vi "convert V to d.vi"(8 "error in (no error)":errorcluster, 10 "V_strain (V)":dbl) -> (0 "error out":errorcluster, 1 "C (pF)":dbl, 2 "d (um)":dbl)   [LabVIEW 2019, in "Inst.RP100.lvlib" / "Inst.RP100.lvclass"]
doc: "This VI will convert a voltage applied to the strain cell to expected capacitance and to an expected displacment. Conversion is based on calibration by Razorbill of capacitance vs displacement at 300K, converting the calibration to values at 4K, and by measurements by us of capacitance vs voltage us at 50 mK.\n\nShould be reliable in the range -140 V ... +130 V."
uses:
  Inst.RP100.lvclass
panel:
  out "our measurements <50 mK":cluster{dbl[], dbl[]}[](graph)
  out "convert measured C to expected d":cluster{dbl[], dbl[]}(graph)
  out "calibration from Razorbill":cluster{"all rows":dbl[], "all rows":dbl[]}[](graph)
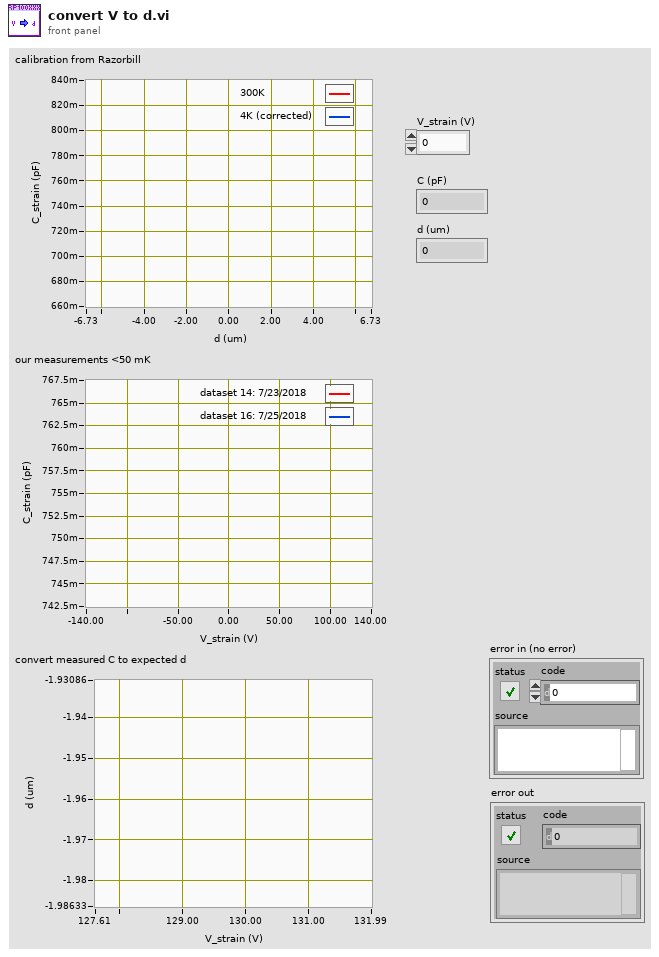
[diagram p1: front panel]
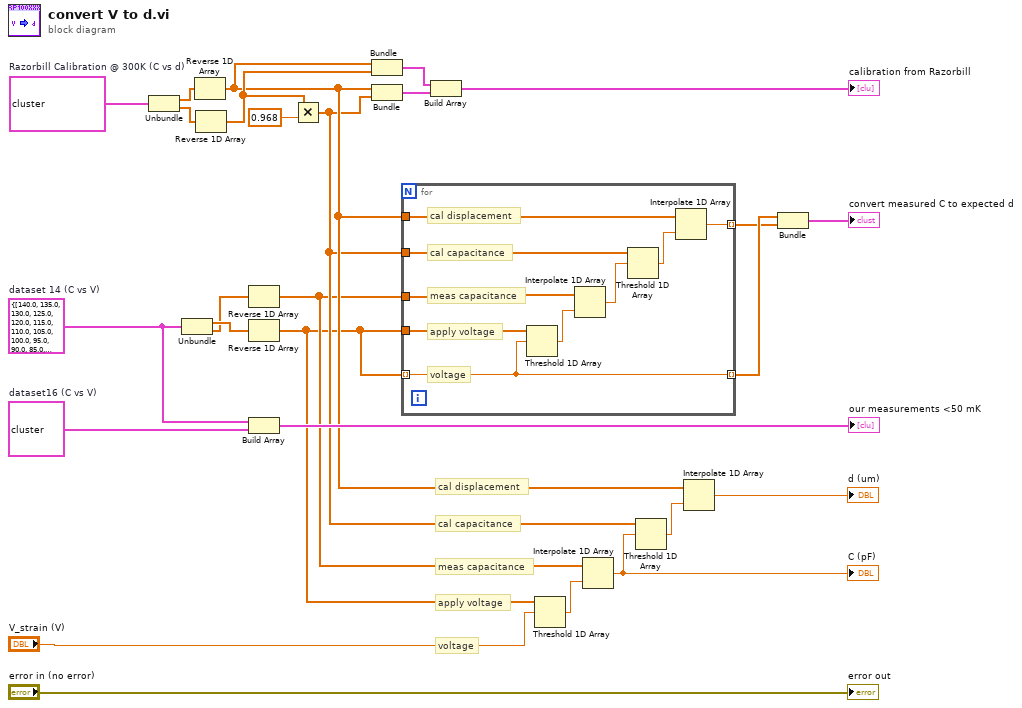
[diagram p0: block diagram]
diagram:
  w18 = cluster{dbl[], dbl[]} {array[987 elements], array[987 elements]}  # dataset16 (C vs V)
  w12 = cluster{dbl[], dbl[]} {[140.0, 135.0, 130.0, 125.0, 120.0, 115.0, 110.0, 105.0, 100.0, 95.0, 90.0, 85.0, 80.0, 75.0, 70.0, 65.0, 60.0, 55.0, 50.0, 45.0, 40.0, 35.0, 30.0, 25.0, 20.0, 15.0, 10.0, 5.0, 0.0, -5.0, -10.0, -15.0, -20.0, -25.0, -30.0, -35.0, -40.0, -45.0, -50.0, -55.0, -60.0, -65.0, -70.0, -75.0, -80.0, -85.0, -90.0, -95.0, -100.0, -105.0, -110.0, -115.0, -120.0, -125.0, -130.0, -135.0, -140.0], [0.75086, 0.74594, 0.74364, 0.74399, 0.74427, 0.74472, 0.74509, 0.74541, 0.74575, 0.746, 0.74625, 0.74658, 0.74691, 0.7473, 0.74773, 0.74809, 0.74842, 0.74876, 0.74909, 0.74944, 0.74978, 0.75017, 0.7506, 0.75099, 0.75141, 0.75177, 0.75204, 0.75244, 0.75278, 0.75325, 0.75365, 0.75411, 0.75455, 0.75494, 0.7553, 0.75566, 0.75599, 0.75638, 0.75685, 0.75732, 0.75778, 0.75825, 0.75871, 0.75909, 0.75947, 0.75987, 0.76027, 0.76073, 0.76126, 0.7618, 0.76235, 0.76284, 0.76328, 0.76376, 0.7642, 0.76462, 0.76508]}  # dataset 14 (C vs V)
  w24 = cluster{"all rows":dbl[], "all rows":dbl[]} {"all rows"=[-6.729466796998171, -6.6508615753295075, -6.562134809022304, -6.484100964873558, -6.406230371444788, -6.327053772256207, -6.245428412267978, -6.164619305879633, -6.075647663492464, -5.989328845304913, -5.9083156755165955, -5.831383773727691, -5.741916548797737, -5.656093313152971, -5.573161947404931, -5.487210443337327, -5.407135965188876, -5.323572002900927, -5.260210317210065, -5.171136643122911, -5.101740511175776, -5.011486184560221, -4.930851989657564, -4.843104727670219, -4.763928128481638, -4.679854007693763, -4.589599681078207, -4.489585293561203, -4.405103045973387, -4.322334930945324, -4.245373877242137, -4.141126631771457, -4.0492981017847, -3.9599183325975904, -3.8688244308507285, -3.7909538374219585, -3.697084673435496, -3.6146430598473858, -3.5308954404994637, -3.4603711294696344, -3.379562023081289, -3.2816115910954142, -3.1942724559080116, -3.111947449977026, -3.0195941855332027, -2.9417235921044327, -2.849813436757688, -2.7673718231695776, -2.691949990540455, -2.604004495535995, -2.5200469824052467, -2.4404622564167235, -2.36393848142776, -2.2797186010684785, -2.205626095730592, -2.114532193983729, -2.0517214794727874, -1.9682595488848245, -1.8890829496962427, -1.7870512497109576, -1.7036913508229805, -1.6311468121334425, -1.5503377057450969, -1.4621823169578096, -1.3532124613735252, -1.2834227785835903, -1.2004710064955528, -1.1193558050072507, -1.0401792058186707, -0.9678824584005259, -0.8818260074415072, -0.8010169010531616, -0.7172692817052386, -0.6449084000756766, -0.555441175145722, -0.44545683294443883, -0.3574851012171276, -0.28126742132811877, -0.16831832944440883, -0.07832637005738796, 0.0019317651510384337, 0.08347549977927926, 0.1613460932080475, 0.2550111937945392, 0.33602436358285637, 0.41038506653213247, 0.4835330498472974, 0.5771456769880814, 0.6785243740934614, 0.759333480481807, 0.8489581257488812, 0.9337552140109366, 1.0208611338840896, 1.1071799520716414, 1.1873768682600758, 1.268430850728386, 1.3416487986378272, 1.4322529482247592, 1.5235567437544475, 1.6159100081982736, 1.695494734186795, 1.782775565545636, 1.8744991486409806, 1.9575121397490083, 2.041994387336823, 2.113008450526582, 2.1990211736141774, 2.306460553698683, 2.382372138487735, 2.460732484076434, 2.5424598757646475, 2.6208814403733367, 2.7094566167262784, 2.7871173163722194, 2.8826189875584465, 2.9602796872043893, 3.0282327993945906, 3.1316929431796687, 3.2115225452481564, 3.2884136343570685, 3.3746100145046363, 3.4556290146758073, 3.543390852620295, 3.623893863908684, 3.712539004855902, 3.7914590671988044, 3.90335869016838, 3.986004367156461, 4.064670807845117, 4.144867724033551, 4.226595115721764, 4.329836620149731, 4.4111704609951445, 4.494183452103172, 4.574992558491518, 4.679309768556475, 4.7582823043450855, 4.837989468373589, 4.9196381498932436, 4.991002036054379, 5.095293009396482, 5.174659096027893, 5.263863953729313, 5.335883757961785, 5.42618181244876, 5.509439679636754, 5.5902487860251, 5.670323264173552, 5.744520716402851, 5.835124865989785, 5.914301465178367, 5.993559689726936, 6.080000945954469, 6.158667386643124, 6.255821971369111, 6.3156941729204785, 6.413950700006309, 6.49567809169452, 6.576854512202816, 6.655459733871476, 6.732595699060353], "all rows"=[0.8239726046128422, 0.8233546085808581, 0.8220124405329421, 0.821121504950495, 0.8201087172717272, 0.8191494340545165, 0.8182629859430387, 0.8172025620339811, 0.816289534286762, 0.8151667172717272, 0.8141683412785723, 0.8133687084708471, 0.8122323180889517, 0.8110619757975797, 0.8099146675467546, 0.8088083678767877, 0.8081422891089108, 0.8074302310231023, 0.8064992533920058, 0.8054477612761276, 0.8044211598302687, 0.803141195033789, 0.8024719207920792, 0.8011270602615816, 0.8001826202175772, 0.7993811874901775, 0.7979858305830583, 0.7972837139713971, 0.7960217680968097, 0.7950810561056105, 0.7941823290900518, 0.7929995599559956, 0.791969167583425, 0.7909528589658965, 0.7895666446644665, 0.7888343485777148, 0.7875887055372204, 0.7869344134413441, 0.7860358679867987, 0.7850114301430142, 0.7841143674367437, 0.7831616428309497, 0.7820587605427209, 0.7809921232123211, 0.7801618547854785, 0.7793579933993399, 0.7781391272460579, 0.7772174697469747, 0.7763693377337733, 0.7753689768976897, 0.774542591859186, 0.7735318753208653, 0.7730381672167216, 0.7717030583058305, 0.7706902706270626, 0.769913592959296, 0.7691769141914191, 0.7683409069795868, 0.7675179738418286, 0.7665459185918592, 0.7656993399339933, 0.7649476571657166, 0.7637281320132012, 0.763066402640264, 0.7619324532453244, 0.76118166483315, 0.7602509460946094, 0.7592192592592593, 0.7584995379537953, 0.7577761181832469, 0.7566159836555084, 0.7559636853685369, 0.7553095674367436, 0.7545268316831683, 0.7536930127298443, 0.7524911595159516, 0.7516026402640263, 0.7507677117711771, 0.7494978437843784, 0.7486007810781078, 0.7475720160301744, 0.7463821680339462, 0.745556204620462, 0.7449387458745874, 0.7439622031536487, 0.7430681953795379, 0.7422603174603174, 0.7408099273927392, 0.7399338349834983, 0.7389769680968097, 0.7378461254125412, 0.7370898632720415, 0.7363176237623762, 0.7354648316831682, 0.7346054809925437, 0.7339969108910891, 0.7333662486248624, 0.7321080308030803, 0.7311915511551155, 0.7302928241395568, 0.7296226622662266, 0.7287305924878202, 0.7276871815181518, 0.7267644884488449, 0.7260787930221593, 0.725368539787312, 0.7245587238723872, 0.7236156152758133, 0.7229932868842439, 0.722025201320132, 0.7213471617161715, 0.7204361188118812, 0.7197943611504007, 0.7191552663837812, 0.717850447901933, 0.7170560176017602, 0.7166521452145214, 0.7153421488815548, 0.7147632651265126, 0.7141495171739396, 0.7132347634763476, 0.7124181423856671, 0.7118056765676567, 0.7111132252780833, 0.7099043696369637, 0.709133905390539, 0.7082290759075907, 0.7075300660066006, 0.7066174697469747, 0.7059883608360835, 0.7052077997799779, 0.7042430551626591, 0.7035231859185919, 0.7028412629262927, 0.7019822574257426, 0.7010927026035936, 0.7004312321232123, 0.6996149438943894, 0.6989039509665251, 0.6982604180418042, 0.6972157865786579, 0.6964940311173975, 0.6957484205563413, 0.6950954565456545, 0.6943097176384305, 0.6935175064173084, 0.692731602760276, 0.6922194191419142, 0.691411846962474, 0.6907249187140936, 0.6900152079207921, 0.689380196259626, 0.6885364136413641, 0.6878995379537953, 0.6871383938393839, 0.6867034543454344, 0.6857485291529153, 0.6849986468646864, 0.6842938895489549, 0.6839582518251826, 0.6833031595159516]}  # Razorbill Calibration @ 300K (C vs d)
  # "cal displacement"
  # "cal capacitance"
  # "meas capacitance"
  # "apply voltage"
  # "voltage"
  n1 = Unbundle(w24) -> ("all rows"=w21:dbl[], "all rows"=w22:dbl[])
  n2 = Unbundle(w12) -> (w14:dbl[], w13:dbl[])
  n3 = Reverse 1D Array(array=w21) -> (reversed array=w7:dbl[])
  n4 = Reverse 1D Array(array=w22) -> (reversed array=w20:dbl[])
  n5 = Reverse 1D Array(array=w13) -> (reversed array=w5:dbl[])
  n6 = Reverse 1D Array(array=w14) -> (reversed array=w4:dbl[])
  n7 = Build Array(w12, w18) -> (→"our measurements <50 mK":cluster{dbl[], dbl[]}[])
  n8 = Multiply(x=w20, y=0.968) -> (x*y=w6:dbl[])
  n9 = Bundle(w7, w20) -> (w19:cluster{dbl[], dbl[]})  [unwired: 1 in]
  n10 = Bundle(w7, w6) -> (w25:cluster{dbl[], dbl[]})  [unwired: 1 in]
  n11 = for {
    tunnel: w4 -> [w27] mode=indexing
    tunnel: w4 -> [w35]
    tunnel: w5 -> [w33]
    tunnel: w6 -> [w30]
    tunnel: w7 -> [w29]
    tunnel: [w28] -> w16 mode=indexing
    tunnel: [w27] -> w17 mode=indexing
    # "cal displacement"
    # "cal capacitance"
    # "meas capacitance"
    # "apply voltage"
    # "voltage"
    n12 = Threshold 1D Array(2:w27, 3:w35) -> (0:w34:dbl)  [unwired: 1 in]
    n13 = Interpolate 1D Array(1:w34, 2:w33) -> (0:w31:dbl)
    n14 = Threshold 1D Array(2:w31, 3:w30) -> (0:w32:dbl)  [unwired: 1 in]
    n15 = Interpolate 1D Array(1:w32, 2:w29) -> (0:w28:dbl)
  }
  n16 = Build Array(w19, w25) -> (→"calibration from Razorbill":cluster{dbl[], dbl[]}[])
  n17 = Threshold 1D Array(2:"V_strain (V)", 3:w4) -> (0:w10:dbl)  [unwired: 1 in]
  n18 = Interpolate 1D Array(1:w10, 2:w5) -> (0:w1:dbl)
  "C (pF)" <- w1
  n19 = Threshold 1D Array(2:w1, 3:w6) -> (0:w9:dbl)  [unwired: 1 in]
  n20 = Interpolate 1D Array(1:w9, 2:w7) -> (0:→"d (um)":dbl)
  n21 = Bundle(w17, w16) -> (→"convert measured C to expected d":cluster{dbl[], dbl[]})  [unwired: 1 in]
  "error out" <- "error in (no error)"
